vi "Keithley 6514 Send System Command.vi"(0 "Resource In":refnum<visa-resource-name>, 1 "Check For SCPI Errors? (T)":bool=TRUE, 5 "System Command Functions":u16(ring) items=["Return to System Preset Defaults", "Autozero Control", "Line Frequency", "Select Power-On Setup", "Save Setup", "Recall Saved Setup", "Clear Error Message Queue", "Reset TimeStamp to 0 seconds", "Simulate Key Press"], 7 "Line Frequency (60Hz:T)":bool=TRUE, 9 "Power On Settings (Preset:1)":u16(ring)=1 items=["RST", "PReset", "SAV0", "SAV1", "SAV2"], 11 "error in (no error)":T1, 12 "Save/Recall Setup Number (SAV0:0)":u16(ring) items=["SAV0", "SAV1", "SAV2"], 13 "autozero (normal:0)":u16(ring) items=["normal", "disable"], 14 "Simulate Key Press Key (SHIFT key:1)":u16(ring)=1 items=["Not Applicable", "SHIFT key", "V key", "I key", "Ohms key", "Q key", "XFBK key", "ZCHK key", "ZCOR key", "Not Applicable", "Not Applicable", "up arrow key", "AUTO key", "down arrow key", "ENTER key", "right arrow key", "GRD key", "LOCAL key", "AVG key", "MEDN key", "REL key", "LIMIT key", "DIGIT key", "RATE key", "left arrow key", "Not Applicable", "STORE key", "RCLL key", "DELAY key", "DAMP key", "HALT key", "TRIG key", "EXIT key"]) -> (4 "Resource Out (dupl)":refnum<visa-resource-name>, 15 "error out":T1)   [LabVIEW 2009, in "Keithley 6514 LV 2009.lvlib"]
doc: "This VI is used to perform some of the basic system commands. These commands are optional and do not need to be performed for any specified type of measurement.\n\nSystem Command Functions:\n0 = Return to System Preset Defaults\n1 = Autozero Control\n2 = Line Frequency\n3 = Power-On Setup\n4 = Save Setup\n5 = Recall Saved Setup\n6 = Clear Error Message Queue\n7 = Reset TimeStamp to 0 seconds\n8 = Simulate Key Press\n\nLine Frequency:\n50 Hz = FALSE\n60 Hz = TRUE\n\nautozero:\n0 = normal\n1 = off\n\nPower On Settings:\n0 = RST\n1 = PRESET\n2 = SAV0\n3 = SAV1\n4 = SAV2\n\nSetup number:\n0 = SAV0\n1 = SAV1\n2 = SAV2\n\nSimulate Key PRess #'s:\n1 = SHIFT key\n2 = V key\n3 = I key\n4 = Ohms key\n5 = Q key\n6 = XFBK key\n7 = ZCHK key\n8 = ZCOR key\n11 = up arrow key\n12 = AUTO key\n13 = down arrow key\n14 = ENTER key\n15 = right arrow key\n16 = GRD key\n17 = LOCAL key\n18 = AVG key\n19 = MEDN key\n20 = REL key\n21 = LIMIT key\n22 = DIGIT key\n23 = RATE key\n24 = left arrow key\n26 = STORE key\n27 = RCLL key\n28 = DELAY key\n29 = DAMP key\n30 = HALT key\n31 = TRIG key\n32 = EXIT key"
uses:
  Keithley 6514 LV 2009.lvlib
panel:
  # "60 Hz\n50 Hz"
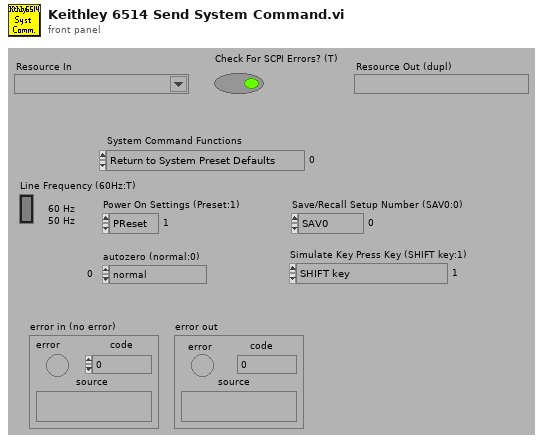
[diagram p1: front panel]
types:
  T1 = cluster{"error":bool, "code":i32, "source":string}
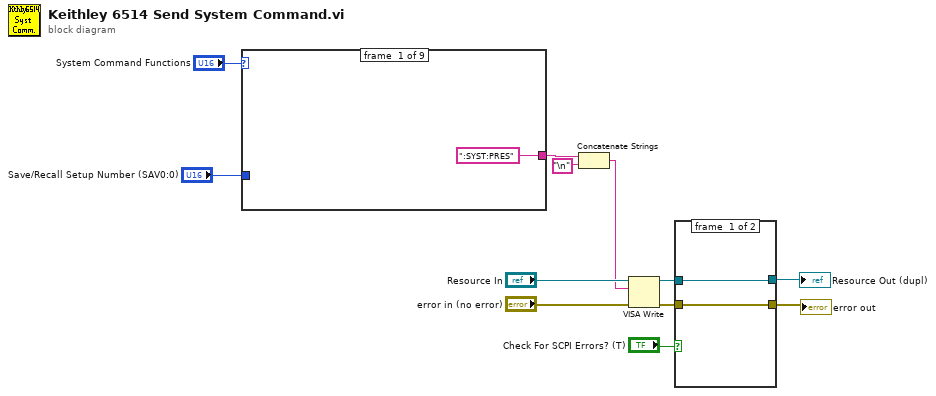
[diagram p0: block diagram]
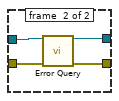
[diagram p2: hidden frame]
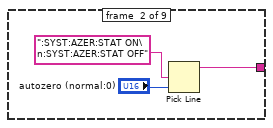
[diagram p3: hidden frame]
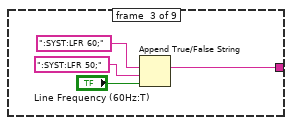
[diagram p4: hidden frame]
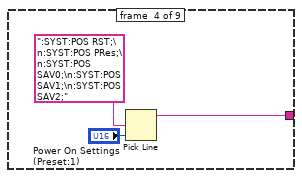
[diagram p5: hidden frame]
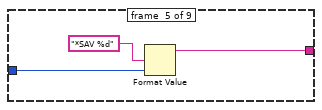
[diagram p6: hidden frame]
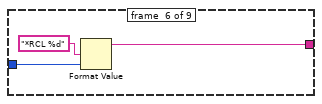
[diagram p7: hidden frame]
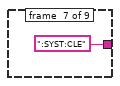
[diagram p8: hidden frame]
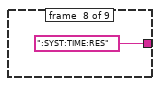
[diagram p9: hidden frame]
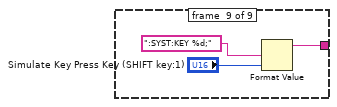
[diagram p10: hidden frame]
diagram:
  n1 = case shown="0, Default" "System Command Functions" {
    tunnel: [":SYST:PRES" w14 w17 w21 w25 w28 ":SYST:CLE" ":SYST:TIME:RES" w32] -> w8
    tunnel: "Save/Recall Setup Number (SAV0:0)" -> [_ _ _ _ w24 w27 _ _ _]
    frame #0 {
    }
    frame #1 {
      n2 = Pick Line(multi-line string=":SYST:AZER:STAT ON\n:SYST:AZER:STAT OFF", line index="autozero (normal:0)") -> (output string=w14:string)  [unwired: 1 in]
    }
    frame #2 {
      n3 = Append True/False String(1:"Line Frequency (60Hz:T)", 2:":SYST:LFR 50;", 3:":SYST:LFR 60;") -> (0:w17:string)  [unwired: 1 in]
    }
    frame #3 {
      n4 = Pick Line(multi-line string=":SYST:POS RST;\n:SYST:POS PRes;\n:SYST:POS SAV0;\n:SYST:POS SAV1;\n:SYST:POS SAV2;", line index="Power On Settings (Preset:1)") -> (output string=w21:string)  [unwired: 1 in]
    }
    frame #4 {
      n5 = Format Value(format string="*SAV %d", value (0)=w24) -> (output string=w25:string)  [unwired: 1 in]
    }
    frame #5 {
      n6 = Format Value(format string="*RCL %d", value (0)=w27) -> (output string=w28:string)  [unwired: 1 in]
    }
    frame #6 {
    }
    frame #7 {
    }
    frame #8 {
      n7 = Format Value(format string=":SYST:KEY %d;", value (0)="Simulate Key Press Key (SHIFT key:1)") -> (output string=w32:string)  [unwired: 1 in]
    }
  }
  n8 = Concatenate Strings(w8, "\n") -> (w6:string)
  n9 = VISA Write(VISA resource name="Resource In", write buffer=w6, error in (no error)="error in (no error)") -> (VISA resource name out=w4:refnum<visa-resource-name>, error out=w3:errorcluster)  [unwired: 1 out]
  n10 = case shown="False" "Check For SCPI Errors? (T)" {
    tunnel: w4 -> [w36 w40]
    tunnel: w3 -> [w35 w39]
    tunnel: [w35 w38] -> w2
    tunnel: [w36 w37] -> w1
    frame #0 {
    }
    frame #1 {
      n11 = call "Error Query.vi"("VISA Resource In"=w40, "error in (no error)"=w39) -> ("VISA Resource Out (dupl)"=w37:refnum<visa-resource-name>, "error out"=w38:errorcluster)  [unwired: 10 in, 2 out]
    }
  }
  "error out" <- w2
  "Resource Out (dupl)" <- w1
